vi "Translator.File.Read.FPsingle.vi"(8 "error in":errorcluster, 10 "Language":string="English") -> (0 "error out":errorcluster)   [LabVIEW 2010]
uses:
  Translator.Control.Fglb.Action.vi
  Translator.Global.vi
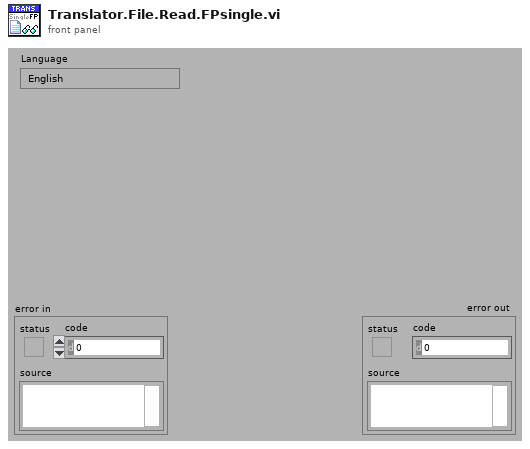
[diagram p1: front panel]
types:
  T1 = typedef "Translator.Control.Fglb.Action.vi" = enum16{"init", "set", "get", "clear"}
  T2 = typedef "Translator.ControlData.ctl" = cluster{"ref":refnum<vi>, "strict?":bool, "ignore?":bool, "type":T3, "root":string, "label":string, "caption":string, "bln.false":string, "bln.true":string, "cols":string[], "rows":string[]}
  T3 = typedef "Translator.ControlTypes.ctl" = enum16{"Cluster", "Array", "Boolean", "Ring", "String", "Tab", "Listbox", "Multicolumn listbox", "Table", "Other"}
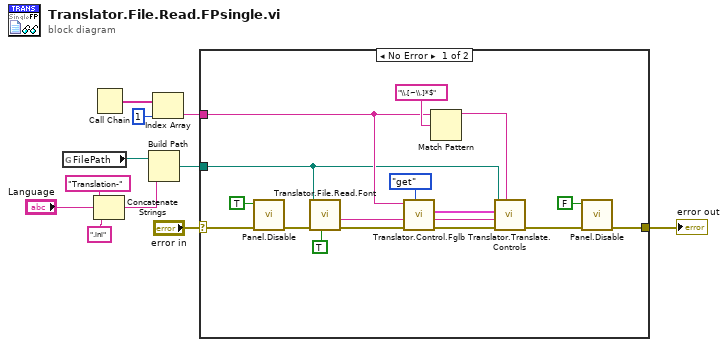
[diagram p0: block diagram]
diagram:
  n1 = global read "Translator.Global.vi" "FilePath"() -> (w2:path)
  n2 = Concatenate Strings("Translation-" ("string"), "Language", ".ini" ("string")) -> (w4:string)
  n3 = Call Chain() -> (call chain=w9:string[])
  n4 = Build Path(base path=w2, name or relative path=w4) -> (appended path=w1:path)
  n5 = Index Array(array=w9, index=1) -> (element=w7:string)
  n6 = case shown="No Error" "error in" {
    selector: "error in" -> [w21 w28]
    tunnel: w1 -> [w14 _]
    tunnel: [w17 w28] -> w11
    tunnel: w7 -> [w22 _]
    frame No Error {
      n7 = call "Panel.Disable.vi"("error in (no error)"=w21, "Defer Panel Updates (F)"=TRUE) -> ("error out"=w15:errorcluster)  [unwired: 9 in]
      n8 = call "Translator.File.Read.Font.vi"("Do not save font? (F)"=TRUE, "error in"=w15, "Translation file"=w14) -> ("error out"=w16:errorcluster, "font name"=w13:string)  [unwired: 6 in, 1 out]
      n9 = call "Translator.Control.Fglb.vi"("Action"=Translator.Control.Fglb.Action.vi."get", "error in (no error)"=w16, "VI name"=w22) -> ("error out"=w23:errorcluster, "Controls out"=w24:T2[])  [unwired: 7 in]
      n10 = Match Pattern(string=w22, regular expression="\\.[~\\.]*$") -> (before substring=w26:string)  [unwired: 4 out]
      n11 = call "Translator.Translate.Controls.vi"("group"=w26, "error in"=w23, "font name"=w13, "Controls out"=w24, "Translation file"=w14) -> ("error out"=w18:errorcluster)  [unwired: 6 in]
      n12 = call "Panel.Disable.vi"("error in (no error)"=w18, "Defer Panel Updates (F)"=FALSE) -> ("error out"=w17:errorcluster)  [unwired: 9 in]
    }
    frame Error {
    }
  }
  "error out" <- w11
